vi "ReportDialog.vi"(8 "error in (no error)":errorcluster) -> (0 "error out":errorcluster, 2 "End time":timestamp=timestamp(3563391600 s since 1904-01-01), 3 "Start time":timestamp=timestamp(3565205999.4435735 s since 1904-01-01))   [LabVIEW 2015]
panel:
  in  "End report":timestamp format="%<%x>T"
  in  "Start report":timestamp format="%<%x>T"
  in  "OK":bool
  # "Select report range"
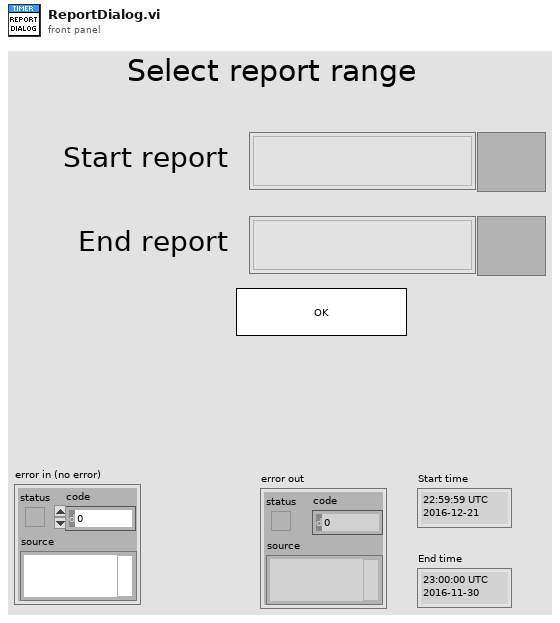
[diagram p1: front panel]
types:
  T1 = typedef "LVDateTimeRec.ctl" = cluster{"fractional second":dbl, "second":i32, "minute":i32, "hour":i32, "day of month":i32, "month":i32, "year":i32, "day of week":i32, "day of year":i32, "DST":i32}
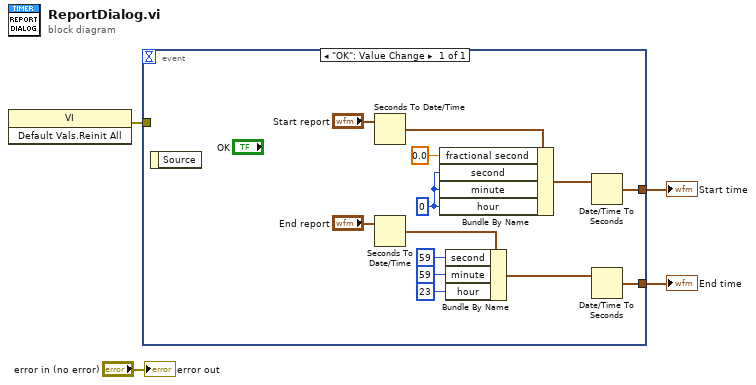
[diagram p0: block diagram]
diagram:
  n1 = invoke class="VI" method="Default Vals.Reinit All"() -> (error out=w3:errorcluster)  [unwired: 3 in, 2 out]
  n2 = event shown="[0] \"OK\": Value Change" {
    selector: _ -> [_]
    dyn-events: _ -> [_]
    timeout: _ -> [_]
    tunnel: [w13] -> w2
    tunnel: [w9] -> w1
    tunnel: w3 -> [_]
    event "OK": Value Change {
      w14 = 0 ("second")
      n3 = event-data() -> ()  [unwired: 1 in, 1 out]
      n4 = Seconds To Date/Time(time stamp (now)="Start report") -> (date time rec=w5:T1)  [unwired: 1 in]
      n5 = Seconds To Date/Time(time stamp (now)="End report") -> (date time rec=w11:T1)  [unwired: 1 in]
      n6 = Bundle By Name(cluster=w5, "fractional second"=0.0, "second"=w14, "minute"=w14, "hour"=w14) -> (w16:T1)
      n7 = Bundle By Name(cluster=w11, "second"=59, "minute"=59, "hour"=23) -> (w10:T1)
      n8 = Date/Time To Seconds(2:w16) -> (0:w13:timestamp)  [unwired: 1 in]
      n9 = Date/Time To Seconds(2:w10) -> (0:w9:timestamp)  [unwired: 1 in]
    }
  }
  "Start time" <- w2
  "End time" <- w1
  "error out" <- "error in (no error)"
